vi "Simulated IO.vi"(0 "sim I/O info in":T1, 9 "data from node input terminals":variant[](array[variant]), 11 "input from node terminal error in":errorcluster) -> (4 "sim I/O info out":T1, 10 "data to node output terminals":variant[](array[variant]), 15 "output to node terminal error out":errorcluster)   [LabVIEW 2010]
uses:
  <vilib>/FPGA/viExecutionOnDevComputer/simIO/customVI/Sim IO Info.ctl
  <vilib>/rvi/customViForEmulation/niLvFPGAUserSpecifiedEmulationVISupport.lvclass
  <vilib>/FPGA/viExecutionOnDevComputer/simIO/customVI/niFPGA Simulated IO.lvlib
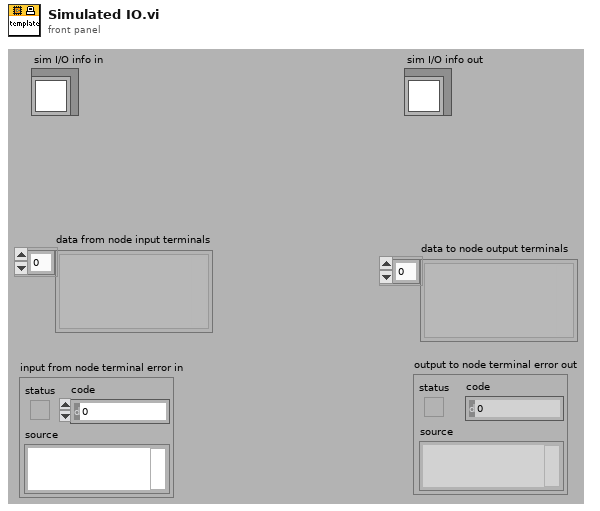
[diagram p1: front panel]
types:
  T1 = typedef "niFPGA Simulated IO.lvlib/Sim IO Info.ctl" = refnum<class "niLvFPGAUserSpecifiedEmulationVISupport.lvclass">
  T2 = typedef "niFPGA Simulated IO.lvlib/Execution Stage.ctl" = enum16{"Initializing", "Running", "Shutting Down"}
  T3 = typedef "niFPGA Simulated IO.lvlib/Node or Element Type.ctl" = enum16{"Read I/O", "Write I/O", "Method", "Read Property", "Write Property"}
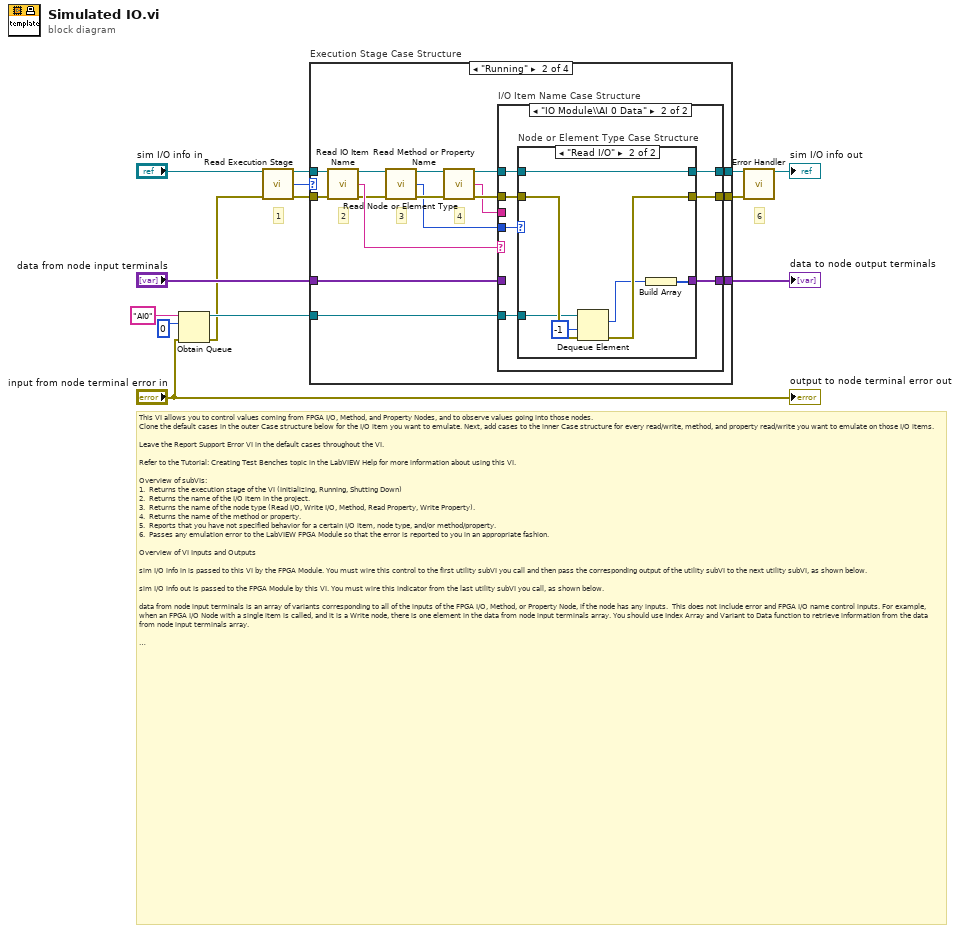
[diagram p0: block diagram]
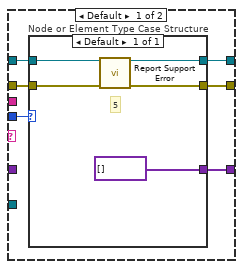
[diagram p3: hidden frame]
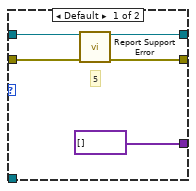
[diagram p4: hidden frame]
diagram:
  # "1"
  # "6"
  # "This VI allows you to control values coming from FPGA I/O, Method, and Property Nodes, and to observe values going into those nodes.\nClone the default cases in the outer Case structure below for the I/O item you want to emulate. Next, add cases to the inner Case structure for every read/write, method, and property read/write you want to emulate on those I/O items.  \n\nLeave the Report Support Error VI in the default cases throughout the VI.\n\nRefer to the Tutorial: Creating Test Benches topic in the LabVIEW Help for more information about using this VI.\n\nOverview of subVIs:\n1.  Returns the execution stage of the VI (Initializing, Running, Shutting Down)\n2.  Returns the name of the I/O item in the project.\n3.  Returns the name of the node type (Read I/O, Write I/O, Method, Read Property, Write Property).\n4.  Returns the name of the method or property.\n5.  Reports that you have not specified behavior for a certain I/O item, node type, and/or method/property.\n6.  Passes any emulation error to the LabVIEW FPGA Module so that the error is reported to you in an appropriate fashion.\n\nOverview of VI Inputs and Outputs\n\nsim I/O info in is passed to this VI by the FPGA Module. You must wire this control to the first utility subVI you call and then pass the corresponding output of the utility subVI to the next utility subVI, as shown below.\n\nsim I/O info out is passed to the FPGA Module by this VI. You must wire this indicator from the last utility subVI you call, as shown below.\n\ndata from node input terminals is an array of variants corresponding to all of the inputs of the FPGA I/O, Method, or Property Node, if the node has any inputs.  This does not include error and FPGA I/O name control inputs. For example, when an FPGA I/O Node with a single item is called, and it is a Write node, there is one element in the data from node input terminals array. You should use Index Array and Variant to Data function to retrieve information from the data from node input terminals array.\n\ndata to node output terminals is an array of variants corresponding to all the outputs of the FPGA I/O, Method, or Property Node, if the node has any outputs.  This does not include error and FPGA I/O name control outputs. For example, when an FPGA I/O node with a single item is called, and it is a Read node, there should be one element in the data to node output terminals array. You should use To Variant and Build Array functions to pass the information to the data to node output terminals array.\n\ninput from node terminal error in is the error that gets passed into the FPGA I/O, Method, or Property Node, if the node is configured so that the error input is shown. If the node is configured so that the error input is not shown, the value of this input corresponds to \"no error\" (status is false, error code is 0). \n\noutput to node terminal error out is the error that gets passed out of the FPGA I/O, Method, or Property Node, if the node is configured so that the error output is shown.  If the node is configured so that the error output is not shown, the value of this output is ignored."
  n1 = Obtain Queue(name (unnamed)="AI0", element data type=i16 0, error in (no error)="input from node terminal error in") -> (queue out=w5:refnum<queue>, error out=w4:errorcluster)  [unwired: 2 in, 1 out]
  n2 = call <vilib>:"Read Execution Stage.vi"("sim I/O info in"="sim I/O info in", "error in (no error)"=w4) -> ("sim I/O info out"=w8:T1, "execution stage"=w6:T2, "error out"=w7:errorcluster)  [unwired: 11 out]
  n3 = case "Execution Stage Case Structure" shown="\"Running\"" w6 {
    tunnel: [_ w31 _ _] -> w13
    tunnel: [w16 w26 w64 w66] -> w9
    tunnel: [w15 w22 w63 w65] -> w11
    tunnel: w8 -> [w15 w20 w63 w65]
    tunnel: w7 -> [w16 w19 w64 w66]
    tunnel: "data from node input terminals" -> [_ w32 _ _]
    tunnel: w5 -> [_ w17 _ _]
    frame "Initializing" {
    }
    frame "Running" {
      # "4"
      # "3"
      # "2"
      n4 = call <vilib>:"Read IO Item Name.vi"("sim I/O info in"=w20, "error in (no error)"=w19) -> ("sim I/O info out"=w21:T1, "I/O item name"=w30:string, "error out"=w29:errorcluster)  [unwired: 11 out]
      n5 = call <vilib>:"Read Node or Element Type.vi"("sim I/O info in"=w21, "error in (no error)"=w29) -> ("sim I/O info out"=w18:T1, "node or element type"=w27:T3, "error out"=w28:errorcluster)  [unwired: 11 out]
      n6 = call <vilib>:"Read Method or Property Name.vi"("sim I/O info in"=w18, "error in (no error)"=w28) -> ("sim I/O info out"=w24:T1, "method or property name"=w23:string, "error out"=w25:errorcluster)  [unwired: 11 out]
      n7 = case "I/O Item Name Case Structure" shown="\"IO Module\\\\AI 0 Data\"" w30 {
        tunnel: w32 -> [_ _]
        tunnel: [w34 w46] -> w31
        tunnel: w25 -> [w38 w50]
        tunnel: [w37 w49] -> w26
        tunnel: w24 -> [w36 w48]
        tunnel: [w35 w47] -> w22
        tunnel: w27 -> [w33 w45]
        tunnel: w23 -> [_ _]
        tunnel: w17 -> [_ w44]
        frame Default {
          n8 = case "Node or Element Type Case Structure" shown="Default" w33 {
            tunnel: w38 -> [w43]
            tunnel: [w42] -> w37
            tunnel: w36 -> [w41]
            tunnel: [w40] -> w35
            tunnel: [variant[] []] -> w34
            frame Default {
              # "5"
              n9 = call <vilib>:"Report Support Error.vi"("sim I/O info in"=w41, "error in (no error)"=w43) -> ("sim I/O info out"=w40:T1, "error out"=w42:errorcluster)  [unwired: 12 out]
            }
          }
        }
        frame "IO Module\\AI 0 Data" {
          n10 = case "Node or Element Type Case Structure" shown="\"Read I/O\"" w45 {
            tunnel: w50 -> [w55 w60]
            tunnel: [w54 w61] -> w49
            tunnel: w48 -> [w53 w62]
            tunnel: [w52 w62] -> w47
            tunnel: [variant[] [] w56] -> w46
            tunnel: w44 -> [_ w59]
            frame Default {
              # "5"
              n11 = call <vilib>:"Report Support Error.vi"("sim I/O info in"=w53, "error in (no error)"=w55) -> ("sim I/O info out"=w52:T1, "error out"=w54:errorcluster)  [unwired: 12 out]
            }
            frame "Read I/O" {
              n12 = Dequeue Element(queue=w59, timeout in ms (-1)=-1, error in (no error)=w60) -> (element=w57:i16, error out=w61:errorcluster)  [unwired: 2 out]
              n13 = Build Array(w57) -> (w56:i16[])
            }
          }
        }
      }
    }
    frame "Shutting Down" {
    }
    frame Default {
    }
  }
  "data to node output terminals" <- w13
  n14 = call <vilib>:"Error Handler.vi"("sim I/O info in"=w11, "error in"=w9) -> ("sim I/O info out"=→"sim I/O info out":T1)  [unwired: 13 out]
  "output to node terminal error out" <- "input from node terminal error in"
